vi "ProvisioningSetEndpointAuthsRoutedMessage_Create.vi"(7 "Header":T2, 8 "error in (no error)":errorcluster, 11 "ProvisioningSetEndpointAuthsRoutedMessage":T1) -> (0 "error out":errorcluster, 3 "Message":T4)   [LabVIEW 2017]
uses:
  <vilib>/addons/InsightCM/MessageBus/Base/controls/Message.ctl
  <vilib>/addons/InsightCM/MessageBus/Base/controls/MessageHeader.ctl
  <vilib>/addons/InsightCM/MessageBus/Base/controls/KeyValuePair.ctl
  <vilib>/addons/InsightCM/MessageBus/MessageLibrary/Provisioning/controls/ProvisioningSetEndpointAuthsRoutedMessageBody.ctl
  <vilib>/addons/InsightCM/MessageBus/Base/controls/MessageClassType.ctl
  <vilib>/addons/InsightCM/Utilities/PropertyHelpers/PropertyHelpers.lvlib
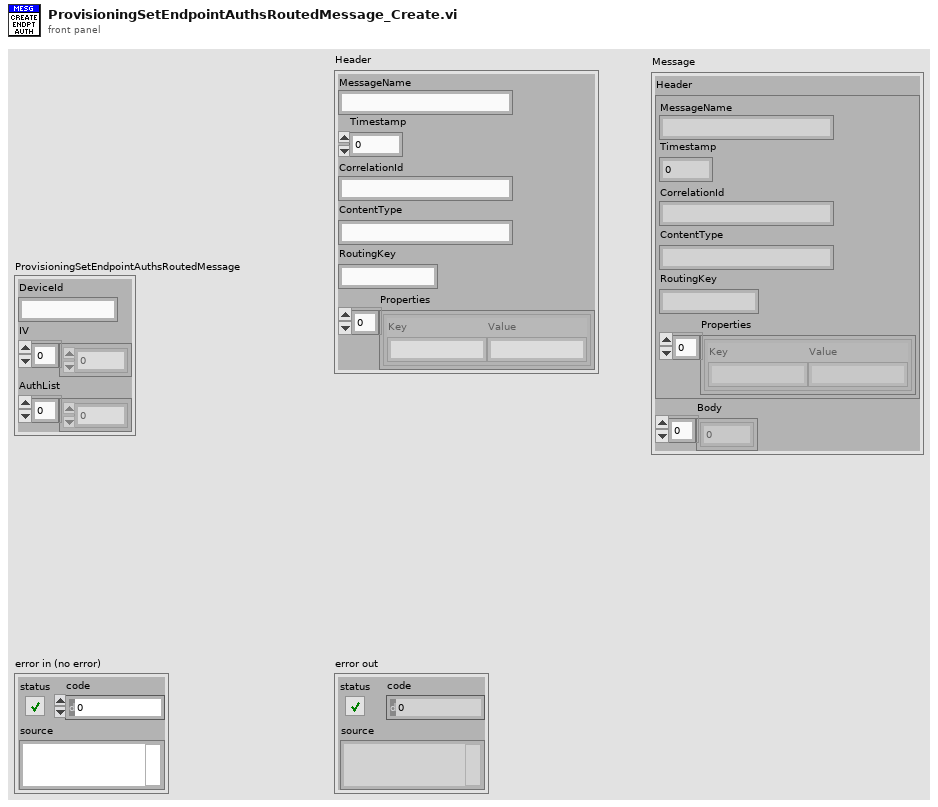
[diagram p1: front panel]
types:
  T1 = typedef "ProvisioningSetEndpointAuthsRoutedMessageBody.ctl" = cluster{"DeviceId":string, "IV":u8[], "AuthList":u8[]}
  T2 = typedef "MessageHeader.ctl" = cluster{"MessageName":string, "Timestamp":i64, "CorrelationId":string, "ContentType":string, "RoutingKey":string, "Properties":T3[]}
  T3 = typedef "KeyValuePair.ctl" = cluster{"Key":string, "Value":string}
  T4 = typedef "Message.ctl" = cluster{"Header":T2, "Body":u8[]}
  T5 = cluster{"DeviceId":string, "IV":string, "AuthList":string}
  T6 = typedef "MessageClassType.ctl" = enum16{"Request", "Response", "Broadcast", "RoutedMessage"}
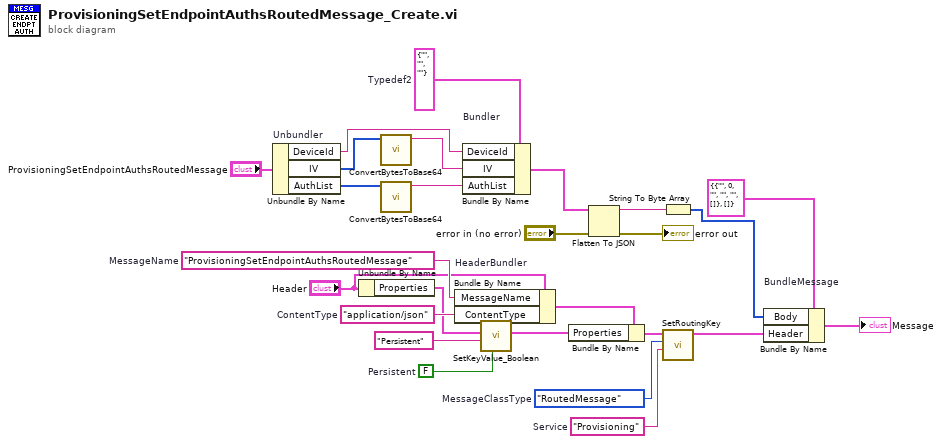
[diagram p0: block diagram]
diagram:
  w6 = T5 {"DeviceId"="", "IV"="", "AuthList"=""}  # Typedef2
  w22 = MessageClassType."RoutedMessage"  # MessageClassType
  w10 = "Provisioning"  # Service
  w17 = FALSE  # Persistent
  w23 = "ProvisioningSetEndpointAuthsRoutedMessage"  # MessageName
  w20 = "application/json"  # ContentType
  n1 = Unbundle By Name "Unbundler"("ProvisioningSetEndpointAuthsRoutedMessage") -> ("DeviceId"=w5:string, "IV"=w4:u8[], "AuthList"=w2:u8[])
  n2 = Unbundle By Name("Header") -> ("Properties"=w19:T3[])
  n3 = call <vilib>:"ConvertBytesToBase64.vi"("U8 array"=w4) -> ("base64 encoded"=w3:string)  [unwired: 10 in]
  n4 = call <vilib>:"ConvertBytesToBase64.vi"("U8 array"=w2) -> ("base64 encoded"=w1:string)  [unwired: 10 in]
  n5 = Bundle By Name "HeaderBundler"(cluster="Header", "MessageName"=w23, "ContentType"=w20) -> (w14:T2)
  n6 = Bundle By Name "Bundler"(cluster=w6, "DeviceId"=w5, "IV"=w3, "AuthList"=w1) -> (w7:T5)
  n7 = call <vilib>:"SetKeyValue_Boolean.vi"("value"=w17, "key"="Persistent" ("Key"), "key value pairs"=w19) -> ("key value pairs out"=w13:T3[])  [unwired: 8 in]
  n8 = Bundle By Name(cluster=w14, "Properties"=w13) -> (w15:T2)
  n9 = Flatten To JSON(anything=w7, error in (no error)="error in (no error)") -> (JSON string=w9:string, 11:→"error out":errorcluster)  [unwired: 1 in]
  n10 = String To Byte Array(string=w9) -> (unsigned byte array=w25:u8[])
  n11 = call <vilib>:"SetRoutingKey.vi"("SendTo"=w10, "MessageClassType"=w22, "Message Header in"=w15) -> ("Message Header out"=w16:T2)  [unwired: 8 in]
  n12 = Bundle By Name "BundleMessage"(cluster=T4 {"Header"={"MessageName"="", "Timestamp"=0, "CorrelationId"="", "ContentType"="", "RoutingKey"="", "Properties"=[]}, "Body"=[]} ("Message"), "Body"=w25, "Header"=w16) -> (→"Message":T4)
